vi "Equip-Get AO Channels.vi"(7 "Outputs":T1[](array[typedef]) items=["--unused--", "Right primary", "Right secondary", "Left primary", "Left secondary", "Shocks", "Startle", "Background", "Shaker", "Blue laser"], 11 "error in (no error)":errorcluster) -> (8 "AO Channels":i32[](array[numeric]), 15 "error out":errorcluster)   [LabVIEW 2020]
uses:
  Type Defs/Output sources.ctl
  <vilib>/Utility/config.llb/Read Key (I32).vi
  <vilib>/Utility/config.llb/NI_LVConfig.lvlib
panel:
  in  "Output sources":T1 items=["--unused--", "Right primary", "Right secondary", "Left primary", "Left secondary", "Shocks", "Startle", "Background", "Shaker", "Blue laser"]
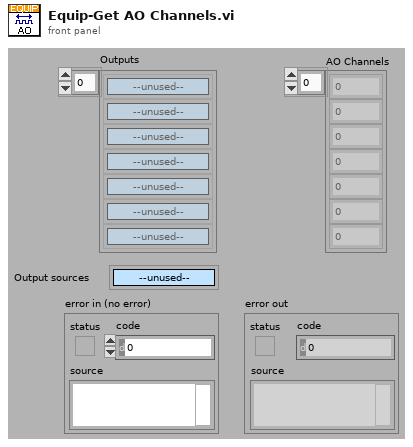
[diagram p1: front panel]
types:
  T1 = typedef "Output sources.ctl" = u16
  T2 = typedef "NI_LVConfig.lvlib/Config Data RefNum.ctl" = refnum<k1>
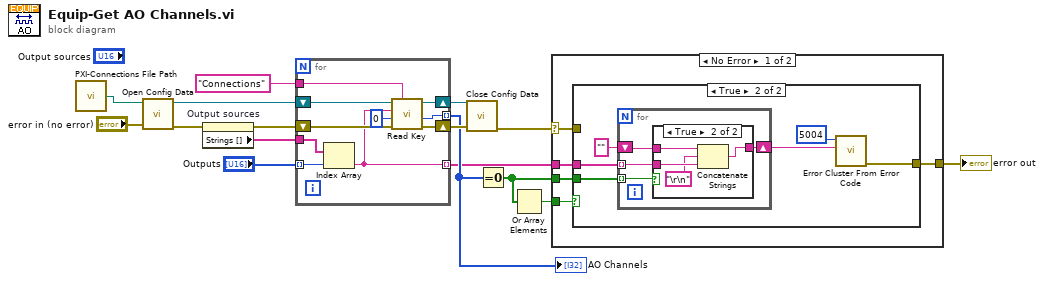
[diagram p0: block diagram]
diagram:
  n1 = call "PXI-Connections File Path.vi"() -> ("Path"=w1:path)  [unwired: 1 in]
  n2 = call <vilib>:"Open Config Data.vi"("error in (no error)"="error in (no error)", "configuration file path"=w1) -> ("error out"=w6:errorcluster, "refnum"=w5:T2)  [unwired: 7 in, 1 out]
  n3 = property on="Output sources" class="Ring (strict)"(error in=w6) -> (error out=w13:errorcluster, "Strings []"=w14:string[])  [unwired: 1 in, 1 out]
  n4 = for {
    tunnel: "Outputs" -> [w25] mode=indexing
    tunnel: w14 -> [w26]
    tunnel: [w21] -> w10 mode=indexing
    shift-right: [w20] -> w12
    shift-left: w13 -> [w24]
    tunnel: "Connections" ("section") -> [w18]
    tunnel: [w17] -> w3 mode=indexing
    shift-right: [w19] -> w11
    shift-left: w5 -> [w23]
    n5 = Index Array(array=w26, index=w25) -> (element=w17:string)
    n6 = call-poly <vilib>:"Read Key.vi"("section"=w18, "error in (no error)"=w24, "default value"=0, "key"=w17, "refnum"=w23) -> ("error out"=w20:errorcluster, "value"=w21:i32, "refnum out"=w19:T2)  [unwired: 3 in, 1 out]
  }
  "AO Channels" <- w10
  n7 = call <vilib>:"Close Config Data.vi"("error in (no error)"=w12, "refnum"=w11) -> ("error out"=w7:errorcluster)  [unwired: 8 in, 1 out]
  n8 = Equal To 0?(x=w10) -> (x = 0?=w2:bool[])
  n9 = Or Array Elements(Boolean array=w2) -> (logical OR=w9:bool)
  n10 = case shown="No Error" w7 {
    selector: w7 -> [w29 w48]
    tunnel: w9 -> [w31 _]
    tunnel: [w30 w48] -> w8
    tunnel: w3 -> [w28 _]
    tunnel: w2 -> [w27 _]
    frame No Error {
      n11 = case shown="True" w31 {
        tunnel: w29 -> [w32 _]
        tunnel: [w32 w37] -> w30
        tunnel: w28 -> [_ w38]
        tunnel: w27 -> [_ w34]
        frame False {
        }
        frame True {
          n12 = for {
            tunnel: w38 -> [w41] mode=indexing
            shift-right: [w42] -> w36
            shift-left: "" -> [w40]
            tunnel: w34 -> [w39] mode=indexing
            n13 = case shown="True" w39 {
              tunnel: [w43 w47] -> w42
              tunnel: w41 -> [_ w46]
              tunnel: w40 -> [w43 w44]
              frame False {
              }
              frame True {
                n14 = Concatenate Strings(w44, "\r\n", w46) -> (w47:string)
              }
            }
          }
          n15 = call <vilib>:"Error Cluster From Error Code.vi"("error message (\"\")"=w36, "error code (0)"=5004) -> ("error out"=w37:errorcluster)  [unwired: 7 in]
        }
      }
    }
    frame Error {
    }
  }
  "error out" <- w8
